vi "Resolve Numeric Sign.vi"(8 "error in (no error)":errorcluster, 10 "Numeric String":string, 11 "Alpaca CLI Parser in":refnum<class "JSON Parser.lvclass">) -> (0 "error out":errorcluster, 2 "Negative?":bool, 3 "Alpaca CLI Parser out":refnum<class "JSON Parser.lvclass">)   [LabVIEW 2019, in "JKI JSON Serialization.lvlib" / "JSON Parser.lvclass"]
doc: "JKI JSON 1.1.10.37\nTomi Maila - JKI\nCopyright (c) 2017, JKI"
uses:
  JSON Parser.lvclass
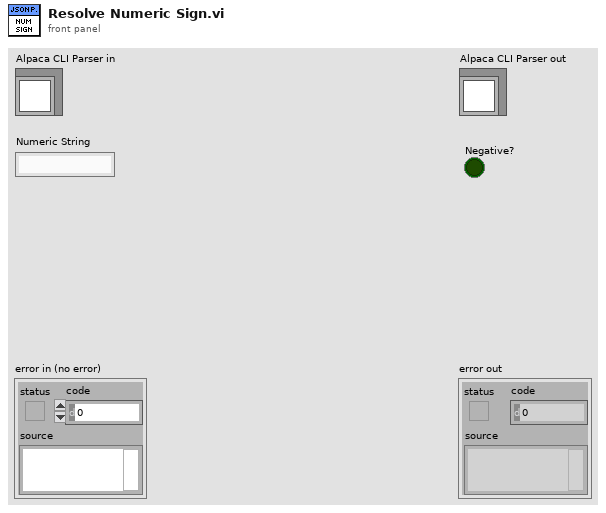
[diagram p1: front panel]
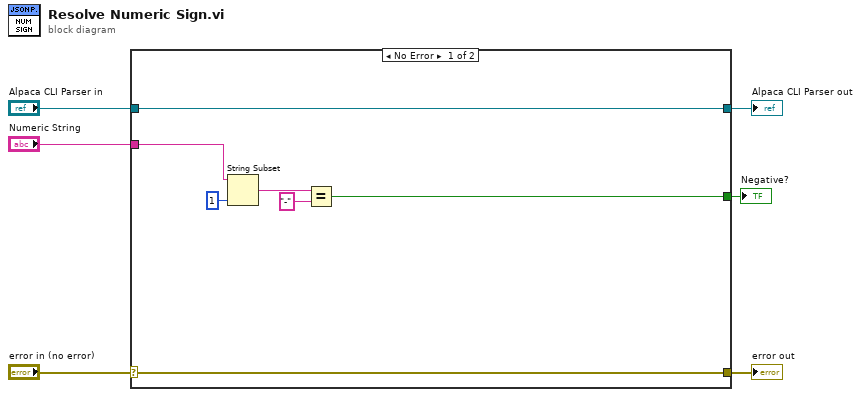
[diagram p0: block diagram]
diagram:
  n1 = case shown="No Error" "error in (no error)" {
    selector: "error in (no error)" -> [w12 w15]
    tunnel: [w12 w15] -> w5
    tunnel: [w13 w14] -> w3
    tunnel: "Alpaca CLI Parser in" -> [w13 w14]
    tunnel: "Numeric String" -> [w11 _]
    tunnel: [w7 _] -> w1
    frame No Error {
      n2 = String Subset(string=w11, length (rest)=1 ("length (rest)")) -> (substring=w9:string)  [unwired: 1 in]
      n3 = Equal?(x=w9, y="-") -> (x = y?=w7:bool)
    }
    frame Error {
    }
  }
  "error out" <- w5
  "Alpaca CLI Parser out" <- w3
  "Negative?" <- w1
